vi "Agilent.vi"() -> ()   [LabVIEW 2022 SP3]
uses:
  Pulsers/PulserGlobals.vi
panel:
  in  "Modify Arb":bool
  in  "Trigger Source":T1={"Trigger Source"=TRUE, "Trigger In\nSlope"=TRUE}
  in  "Burst Settings":T2={"Burst Mode"=0, "Trigger"=0, "Burst Rate (Hz)"=100.0, "Burst Phase (deg)"=0, "Burst Count "=1, "Gated Polarity"=FALSE} {"Burst Count" min=1 max=50000; "Burst Phase (deg)" min=-360 max=360; "Burst Rate (Hz)" min=0.002 max=1000000.0 format="%.2f"; "Trigger" items=["Int", "Ext", "Bus"]; "Burst Mode" items=["Off", "Triggered", "Ext gated"]}
  in  "Select Arb":bool
  in  "Instrument Resource Name":refnum<visa-resource-name>="GPIB::10::INSTR"
  in  "Arb Waves In Mem":u16(ring)
  in  "Arb Wave Op":u16(ring) items=["Copy wfm from volatile", "Delete wfm from volatile", "Delete one wfm from non-volatile", "Delete all wfms from non-volatile"]
  in  "Query Arb Wvs":bool
  in  "Enable Output":bool
  in  "Exit Program":bool
  in  "Duty Cycle (50 %)":i32=50 min=20 max=80
  in  "Basic Wvfrm":T3={"Waveform Shape"=1, "Freq or Time"=1000.0, "Amplitude (Vpp)"=0.1, "Offset (V)"=0.0, "Time int Type"=0} {"Time int Type" items=["Frequency", "Period"]; "Offset (V)" min=-10.0 max=10.0 format="%.2f"; "Amplitude (Vpp)" min=0.001 max=20.0 format="%.2f"; "Freq or Time" min=1e-06 max=80000000.0 format="%^#.2e"; "Waveform Shape" items=["DC"=0, "Sine"=1, "Square"=2, "Triangle"=3, "Ramp"=4, "Pulse"=6, "Noise"=7, "Sinc"=8, "Neg. Ramp"=9, "Exp. Rise"=10, "Exp. Fall"=11, "Cardiac"=12, "Volatile"=13]}
  out "dup VISA session":refnum<visa-resource-name>
  in  "error in (no error)":errorcluster
  out "error out":errorcluster
  # "Select on of Arb waves in pull down menu and then click Select Arb to place it on output. Use Modify Arb to carry out one of the actions in the lower pull down menu."
  # "Manage Arb Memory"
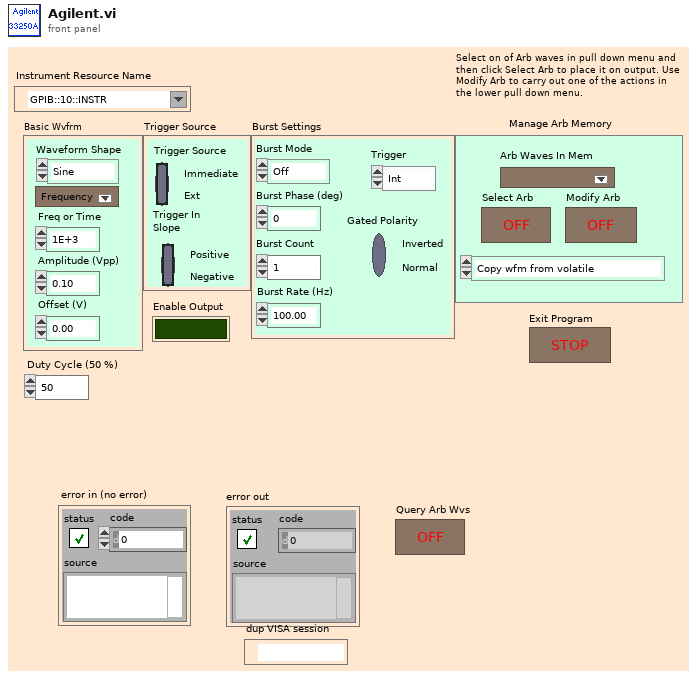
[diagram p1: front panel]
types:
  T1 = cluster{"Trigger Source":bool, "Trigger In\nSlope":bool}
  T2 = cluster{"Burst Mode":u16, "Trigger":u16, "Burst Rate (Hz)":dbl, "Burst Phase (deg)":i32, "Burst Count ":i32, "Gated Polarity":bool}
  T3 = cluster{"Waveform Shape":u16, "Freq or Time":dbl, "Amplitude (Vpp)":dbl, "Offset (V)":dbl, "Time int Type":u16}
  T4 = cluster{"Therapy frequency (MHz)":dbl, "Therapy amplitude (mV)":dbl, "time therapy on (s)":dbl, "Therapy Delay (ms) ":dbl, "Time (s)":dbl}
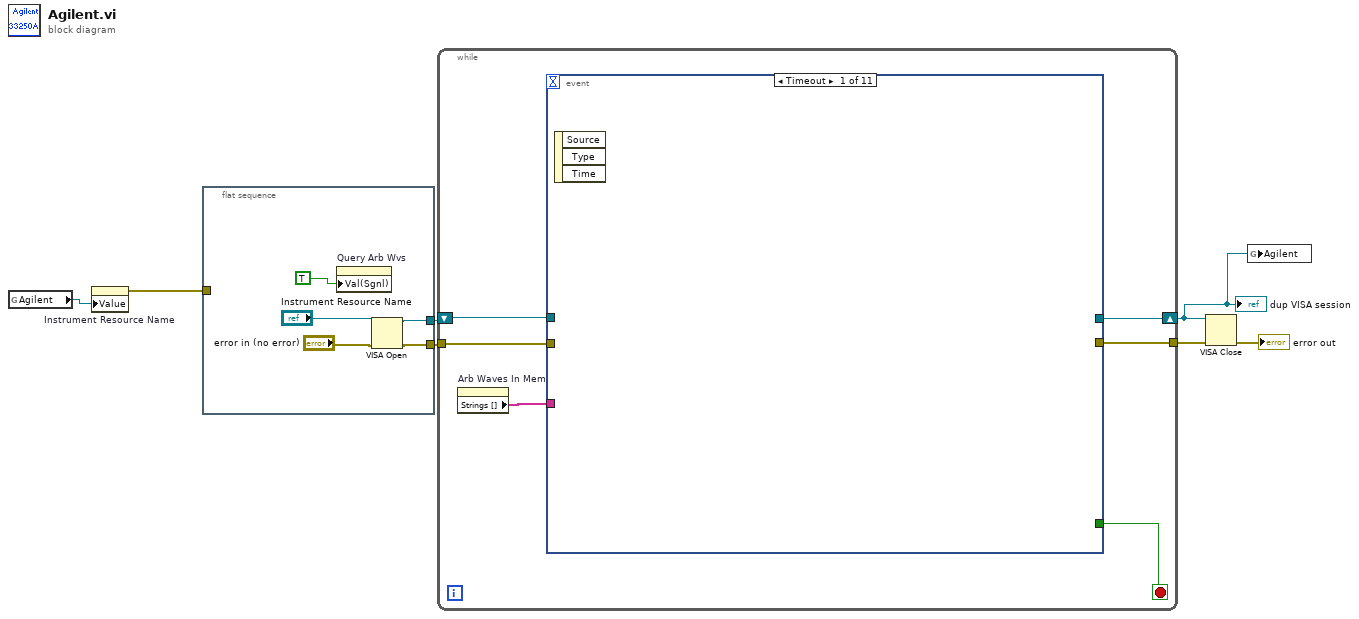
[diagram p0: block diagram]
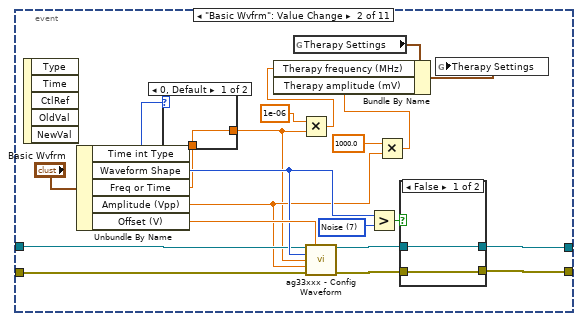
[diagram p2: hidden frame]
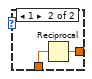
[diagram p3: hidden frame]
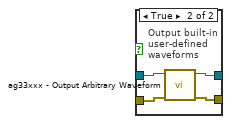
[diagram p4: hidden frame]
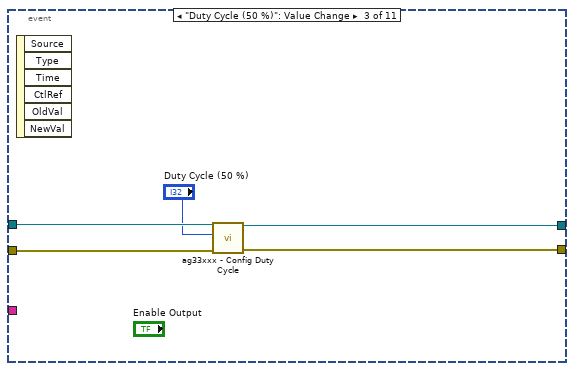
[diagram p5: hidden frame]
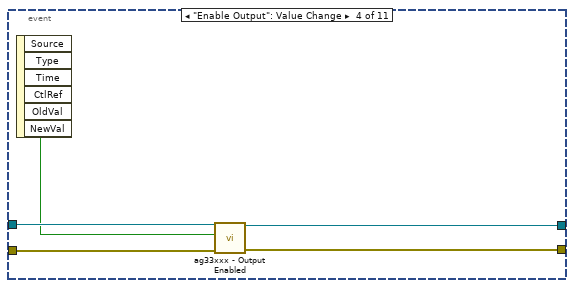
[diagram p6: hidden frame]
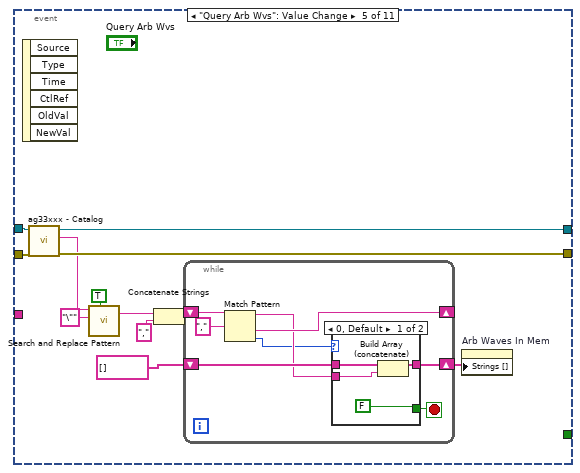
[diagram p7: hidden frame]
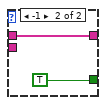
[diagram p8: hidden frame]
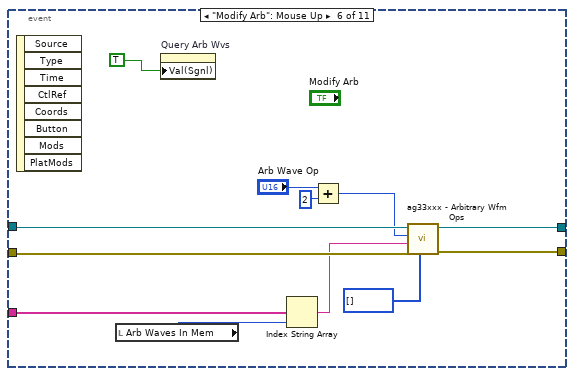
[diagram p9: hidden frame]
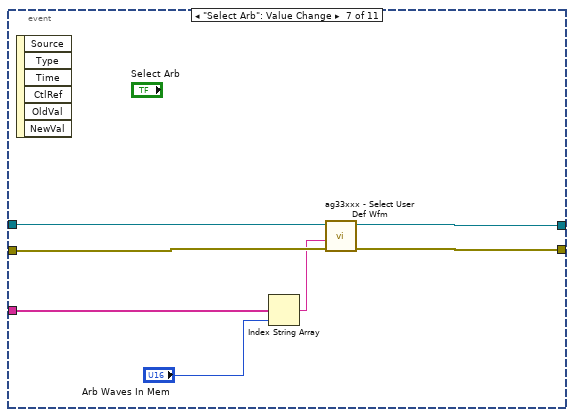
[diagram p10: hidden frame]
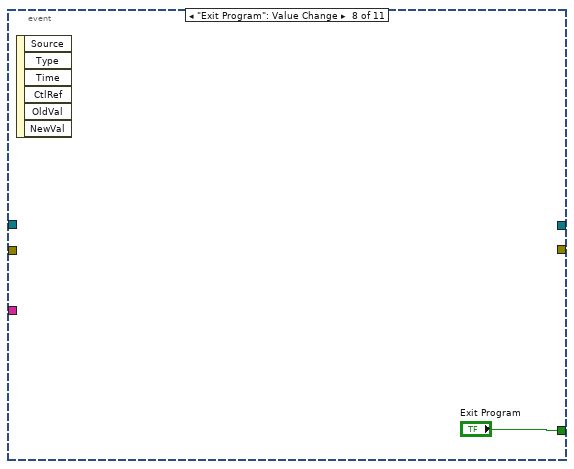
[diagram p11: hidden frame]
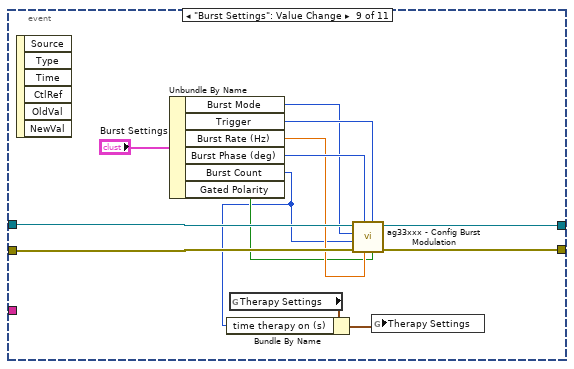
[diagram p12: hidden frame]
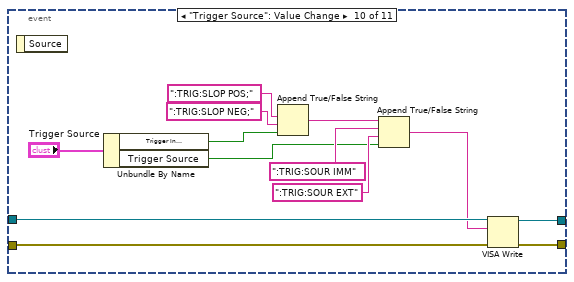
[diagram p13: hidden frame]
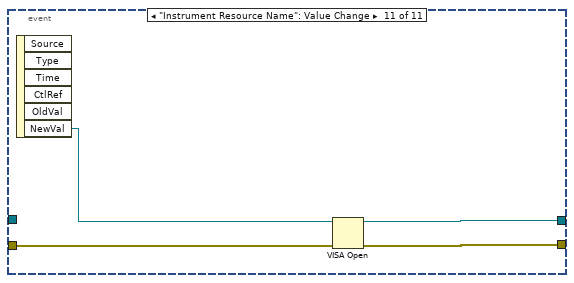
[diagram p14: hidden frame]
diagram:
  n1 = global read "PulserGlobals.vi" "Agilent"() -> (w3:refnum<visa-resource-name>)
  n2 = property on="Instrument Resource Name" class="VISAName"("Value"=w3) -> (error out=w2:errorcluster)  [unwired: 2 in, 1 out]
  n3 = flat-sequence {
    tunnel: [w10] -> w7
    tunnel: [w9] -> w6
    tunnel: w2 -> [_]
    frame #0 {
      n4 = property on="Query Arb Wvs" class="Bool (strict)"("Val(Sgnl)"=TRUE) -> ()  [unwired: 2 in, 2 out]
      n5 = VISA Open(error in (no error)="error in (no error)", VISA resource name="Instrument Resource Name") -> (VISA resource name=w10:refnum<visa-resource-name>, error out=w9:errorcluster)  [unwired: 3 in]
    }
  }
  n6 = while {
    tunnel: w6 -> [w17]
    tunnel: [w16] -> w5
    shift-right: [w13] -> w1
    shift-left: w7 -> [w18]
    stop <- w15 stop-if-true
    n7 = property on="Arb Waves In Mem" class="Ring (strict)"() -> ("Strings []"=w14:string[])  [unwired: 2 in, 2 out]
    n8 = event shown="[0] Timeout" {
      selector: _ -> [_ _ _ _ _ _ _ _ _ _ _]
      dyn-events: _ -> [_ _ _ _ _ _ _ _ _ _ _]
      timeout: _ -> [_ _ _ _ _ _ _ _ _ _ _]
      tunnel: w18 -> [_ w32 w53 w58 w70 w96 w103 _ w117 w120 _]
      tunnel: w17 -> [_ w31 w52 w57 w69 w95 w102 _ w116 w119 w131]
      tunnel: [_ w30 w50 w55 w67 w93 w100 _ w114 w122 w133] -> w13
      tunnel: [_ w29 w49 w56 w68 w94 w101 _ w115 w121 w132] -> w16
      tunnel: [_ _ _ _ _ _ _ "Exit Program" _ _ _] -> w15
      tunnel: w14 -> [_ _ _ _ _ w87 w98 _ _ _ _]
      event Timeout {
        n9 = event-data() -> ()  [unwired: 4 out]
      }
      event "Basic Wvfrm": Value Change {
        w38 = u16 7 items=["DC"=0, "Sine"=1, "Square"=2, "Triangle"=3, "Ramp"=4, "Pulse"=6, "Noise"=7, "Sinc"=8, "Neg. Ramp"=9, "Exp. Rise"=10, "Exp. Fall"=11, "Cardiac"=12, "Volatile"=13] ("Waveform Shape (1: Sine)")
        n10 = event-data() -> ()  [unwired: 6 out]
        n11 = Unbundle By Name("Basic Wvfrm") -> ("Time int Type"=w23:u16, "Waveform Shape"=w35:u16, "Freq or Time"=w25:dbl, "Amplitude (Vpp)"=w26:dbl, "Offset (V)"=w36:dbl)
        n12 = case shown="0, Default" w23 {
          tunnel: [w40 w42] -> w24
          tunnel: w25 -> [w40 w41]
          frame 0, Default {
          }
          frame 1 {
            n13 = Reciprocal(x=w41) -> (1/x=w42:dbl)
          }
        }
        n14 = global read "PulserGlobals.vi" "Therapy Settings"() -> (w22:T4)
        n15 = Multiply(x=1e-06, y=w24) -> (x*y=w19:dbl)
        n16 = call <instrlib>:"ag33xxx - Config Waveform.vi"("VISA session"=w32, "Offset (0.00 V)"=w36, "Waveform Shape (1: Sine)"=w35, "Frequency (1000 Hz)"=w24, "Amplitude (0.1 Vpp)"=w26, "error in (no error)"=w31) -> ("dup VISA session"=w34:refnum<visa-resource-name>, "error out"=w33:errorcluster)  [unwired: 2 in, 6 out]
        n17 = Greater?(x=w35, y=w38) -> (0:w39:bool)
        n18 = Multiply(x=1000.0, y=w26) -> (x*y=w20:dbl)
        n19 = Bundle By Name(cluster=w22, "Therapy frequency (MHz)"=w19, "Therapy amplitude (mV)"=w20) -> (w21:T4)
        n20 = case shown="False" w39 {
          tunnel: [w43 w48] -> w29
          tunnel: [w44 w47] -> w30
          tunnel: w34 -> [w44 w46]
          tunnel: w33 -> [w43 w45]
          frame False {
          }
          frame True {
            # "Output built-in\nuser-defined\nwaveforms"
            n21 = call <instrlib>:"ag33xxx - Output Arbitrary Waveform.vi"("error in (no error)"=w45, "VISA session"=w46) -> ("error out"=w48:errorcluster, "dup VISA session"=w47:refnum<visa-resource-name>)  [unwired: 8 out]
          }
        }
        n22 = global write "PulserGlobals.vi" "Therapy Settings"(w21) -> ()
      }
      event "Duty Cycle (50 %)": Value Change {
        n23 = event-data() -> ()  [unwired: 7 out]
        n24 = call <instrlib>:"ag33xxx - Config Duty Cycle.vi"("error in (no error)"=w52, "Duty Cycle (50 %)"="Duty Cycle (50 %)", "VISA session"=w53) -> ("error out"=w49:errorcluster, "dup VISA session"=w50:refnum<visa-resource-name>)  [unwired: 7 out]
      }
      event "Enable Output": Value Change {
        n25 = event-data() -> ("NewVal"=w54:bool)  [unwired: 6 out]
        n26 = call <instrlib>:"ag33xxx - Output Enabled.vi"("error in (no error)"=w57, "Output Enabled? (T: Yes)"=w54, "VISA session"=w58) -> ("error out"=w56:errorcluster, "dup VISA session"=w55:refnum<visa-resource-name>)  [unwired: 7 out]
      }
      event "Query Arb Wvs": Value Change {
        n27 = event-data() -> ()  [unwired: 7 out]
        n28 = call <instrlib>:"ag33xxx - Catalog.vi"("error in (no error)"=w69, "VISA session"=w70) -> ("error out"=w68:errorcluster, "Catalog"=w64:string, "dup VISA session"=w67:refnum<visa-resource-name>)  [unwired: 1 in, 6 out]
        n29 = call <vilib>:"Search and Replace Pattern.vi"("string"=w64, "regular expression (\"\")"="\"" ("regular expression (\"\")"), "replace all? (F)"=TRUE) -> ("result string"=w61:string)  [unwired: 1 in, 2 out]
        n30 = Concatenate Strings(w61, ",") -> (w59:string)
        n31 = while {
          shift-right: [w76] -> _
          shift-left: w59 -> [w78]
          shift-right: [w74] -> w65
          shift-left: string[] [] -> [w75]
          stop <- w72 stop-if-true
          n32 = Match Pattern(string=w78, regular expression=",") -> (before substring=w73:string, after substring=w76:string, offset past match=w71:i32)  [unwired: 2 out]
          n33 = case shown="0, Default" w71 {
            tunnel: w75 -> [w82 w84]
            tunnel: [w81 w84] -> w74
            tunnel: w73 -> [w80 _]
            tunnel: [FALSE TRUE] -> w72
            frame 0, Default {
              n34 = Build Array (concatenate)(w82, w80) -> (w81:string[])
            }
            frame -1 {
            }
          }
        }
        n35 = property on="Arb Waves In Mem" class="Ring (strict)"("Strings []"=w65) -> ()  [unwired: 2 in, 2 out]
      }
      event "Modify Arb": Mouse Up {
        n36 = event-data() -> ()  [unwired: 9 out]
        n37 = local read "Arb Waves In Mem"() -> (w85:u16)
        n38 = property on="Query Arb Wvs" class="Bool (strict)"("Val(Sgnl)"=TRUE) -> ()  [unwired: 2 in, 2 out]
        n39 = Index String Array(1:w85, 2:w87) -> (0:w88:string)  [unwired: 1 out]
        n40 = Add(x="Arb Wave Op", y=2) -> (x+y=w90:i32)
        n41 = call <instrlib>:"ag33xxx - Arbitrary Wfm Ops.vi"("Data"=i16[] [], "error in (no error)"=w95, "Waveform Name"=w88, "Mode (0: Create wfm & store in volatile)"=w90, "VISA session"=w96) -> ("error out"=w94:errorcluster, "dup VISA session"=w93:refnum<visa-resource-name>)  [unwired: 5 out]
      }
      event "Select Arb": Value Change {
        n42 = event-data() -> ()  [unwired: 7 out]
        n43 = Index String Array(1:"Arb Waves In Mem", 2:w98) -> (0:w99:string)  [unwired: 1 out]
        n44 = call <instrlib>:"ag33xxx - Select User Def Wfm.vi"("error in (no error)"=w102, "User Def. Wfm Name"=w99, "VISA session"=w103) -> ("error out"=w101:errorcluster, "dup VISA session"=w100:refnum<visa-resource-name>)  [unwired: 7 out]
      }
      event "Exit Program": Value Change {
        n45 = event-data() -> ()  [unwired: 7 out]
      }
      event "Burst Settings": Value Change {
        n46 = event-data() -> ()  [unwired: 7 out]
        n47 = Unbundle By Name("Burst Settings") -> ("Burst Mode"=w110:u16, "Trigger"=w111:u16, "Burst Rate (Hz)"=w109:dbl, "Burst Phase (deg)"=w112:i32, "Burst Count"=w105:i32, "Gated Polarity"=w108:bool)
        n48 = global read "PulserGlobals.vi" "Therapy Settings"() -> (w107:T4)
        n49 = Bundle By Name(cluster=w107, "time therapy on (s)"=w105) -> (w106:T4)
        n50 = call <instrlib>:"ag33xxx - Config Burst Modulation.vi"("Gated Polarity (F: Normal)"=w108, "Trigger (0: Int)"=w111, "Burst Rate (100 Hz)"=w109, "Burst Phase (0 deg)"=w112, "error in (no error)"=w116, "Burst Count (1)"=w105, "Burst Mode (0: Off)"=w110, "VISA session"=w117) -> ("error out"=w115:errorcluster, "dup VISA session"=w114:refnum<visa-resource-name>)  [unwired: 2 out]
        n51 = global write "PulserGlobals.vi" "Therapy Settings"(w106) -> ()
      }
      event "Trigger Source": Value Change {
        n52 = event-data() -> ()  [unwired: 2 out]
        n53 = Unbundle By Name("Trigger Source") -> ("Trigger In\nSlope"=w127:bool, "Trigger Source"=w128:bool)
        n54 = Append True/False String(1:w127, 2:":TRIG:SLOP NEG;" ("true string"), 3:":TRIG:SLOP POS;" ("true string")) -> (0:w125:string)  [unwired: 1 out]
        n55 = Append True/False String(1:w128, 2:":TRIG:SOUR EXT", 3:":TRIG:SOUR IMM", 4:w125) -> (0:w118:string)
        n56 = VISA Write(VISA resource name=w120, write buffer=w118, error in (no error)=w119) -> (VISA resource name out=w122:refnum<visa-resource-name>, error out=w121:errorcluster)  [unwired: 1 out]
      }
      event "Instrument Resource Name": Value Change {
        n57 = event-data() -> ("NewVal"=w134:refnum<visa-resource-name>)  [unwired: 6 out]
        n58 = VISA Open(error in (no error)=w131, VISA resource name=w134) -> (VISA resource name=w133:refnum<visa-resource-name>, error out=w132:errorcluster)  [unwired: 3 in]
      }
    }
  }
  "dup VISA session" <- w1
  n59 = VISA Close(VISA resource name=w1, error in (no error)=w5) -> (error out=→"error out":errorcluster)
  n60 = global write "PulserGlobals.vi" "Agilent"(w1) -> ()
